vi "Read HGF_Configuration.vi"(8 "error in (no error)":errorcluster, 11 "HGF_Application in":refnum<class "HGF_Application.lvclass">) -> (0 "error out":errorcluster, 2 "HGF_Configuration":refnum<class "HGF_Configuration.lvclass">, 3 "HGF_Application out":refnum<class "HGF_Application.lvclass">)   [LabVIEW 2012, in "HGF_ApplicationBaseClasses.lvlib" / "HGF_Application.lvclass"]
uses:
  HGF_Application.lvclass
  HGF_Configuration/HGF_Configuration.lvclass
  HGF_Application.lvclass/HGF_Application.ctl
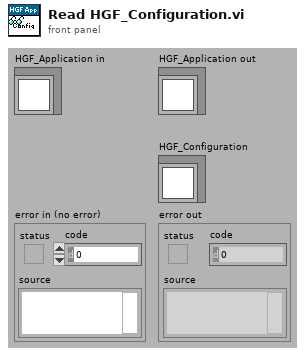
[diagram p1: front panel]
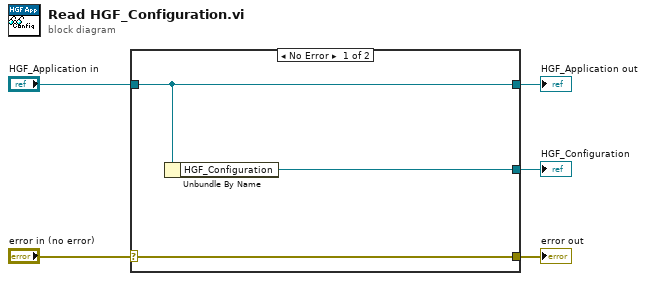
[diagram p0: block diagram]
diagram:
  n1 = case shown="No Error" "error in (no error)" {
    selector: "error in (no error)" -> [w8 w9]
    tunnel: [w8 w9] -> w4
    tunnel: [w7 w10] -> w2
    tunnel: "HGF_Application in" -> [w7 w10]
    tunnel: [w6 _] -> w1
    frame No Error {
      n2 = Unbundle By Name(w7) -> ("HGF_Configuration"=w6:refnum<class "HGF_Configuration.lvclass">)
    }
    frame Error {
    }
  }
  "error out" <- w4
  "HGF_Application out" <- w2
  "HGF_Configuration" <- w1
